vi "InitTableFocus.vi"(8 "error in (no error)":errorcluster, 10 "Focus by Mode":T1, 11 "Instrument in":refnum<class "Instrument.lvclass">) -> (0 "error out":errorcluster, 3 "Instrument out":refnum<class "Instrument.lvclass">)   [LabVIEW 2018, in "Instrument.lvclass"]
uses:
  Instrument.lvclass
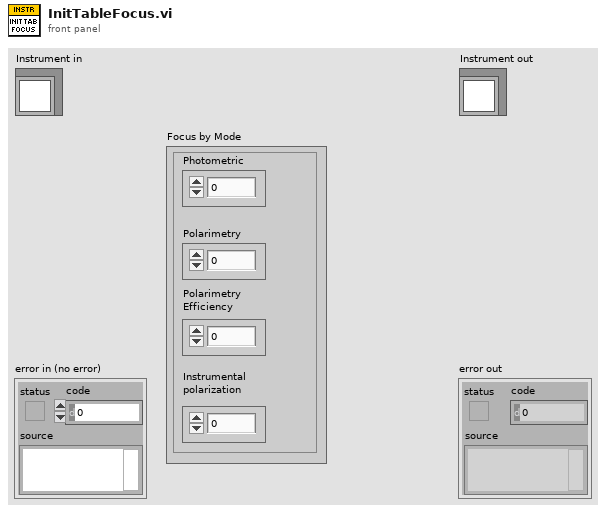
[diagram p1: front panel]
types:
  T1 = cluster{"Photometric":dbl, "Polarimetry":dbl, "Polarimetry \nEfficiency":dbl, "Instrumental  \npolarization":dbl}
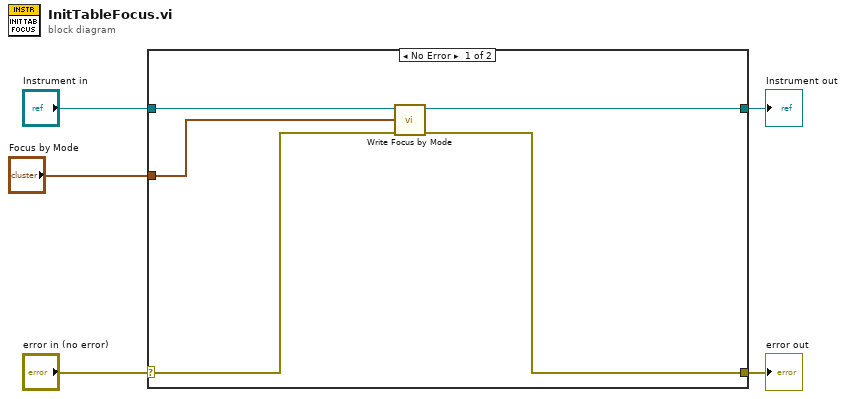
[diagram p0: block diagram]
diagram:
  n1 = case shown="No Error" "error in (no error)" {
    selector: "error in (no error)" -> [w8 w12]
    tunnel: [w7 w12] -> w4
    tunnel: [w9 w11] -> w2
    tunnel: "Instrument in" -> [w10 w11]
    tunnel: "Focus by Mode" -> [w6 _]
    frame No Error {
      n2 = call-dynamic "Write Focus by Mode.vi"("error in (no error)"=w8, "Focus by Mode"=w6, "Instrument in"=w10) -> ("error out"=w7:errorcluster, "Instrument out"=w9:refnum<class "Instrument.lvclass">)  [unwired: 7 in]
    }
    frame Error {
    }
  }
  "error out" <- w4
  "Instrument out" <- w2
